vi "Security System.vi"() -> ()   [LabVIEW 2013]
doc: "This VI simulates the security system by monitoring the\n- Alarm switches\n- Bypass switches, \n-Tamper switches and indicates the corresponding activity with different colours.\nTHe system provides for one indicator light for each zone i.e.\n-Green: Normal\n-Red: Alarm\n-Blue: Bypass\n-Orange: Tamper.\n\n-A bypass input can override an alarm input but can not change the the existing condition of alarm\n-A Tamper input can override both alarm and bypass input but can not change the the existing condition of alarm and bypass.\n-An existing condition can be indicated when an override input is removed."
uses:
  Controls/Security System Indicators.ctl
  Controls/Security States.ctl
  Controls/FGV.ctl
  Controls/Write txt.ctl
panel:
  in  "stop simulation":bool
  out "Zone status indicators":T1
  in  "Tamper":bool[](array[boolean])
  in  "Bypass":bool[](array[boolean])
  in  "Alarm":bool[](array[boolean])
  # "· Green: Normal\n· Red: Alarm\n· Blue: Bypass\n· Orange: Tampe"
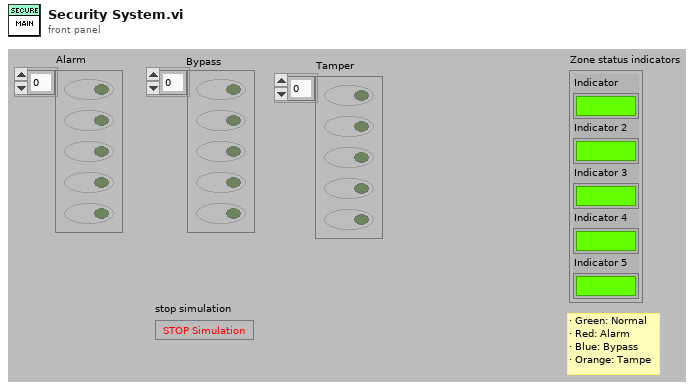
[diagram p1: front panel]
types:
  T1 = typedef "Security System Indicators.ctl" = cluster{"Indicator":bool, "Indicator 2":bool, "Indicator 3":bool, "Indicator 4":bool, "Indicator 5":bool}
  T2 = typedef "Security States.ctl" = enum16{"Initialize", "Main", "Stop"}
  T3 = typedef "Write txt.ctl" = enum16{"Initialize", "Write", "Stop"}
  T4 = typedef "FGV.ctl" = enum16{"Set", "Get"}
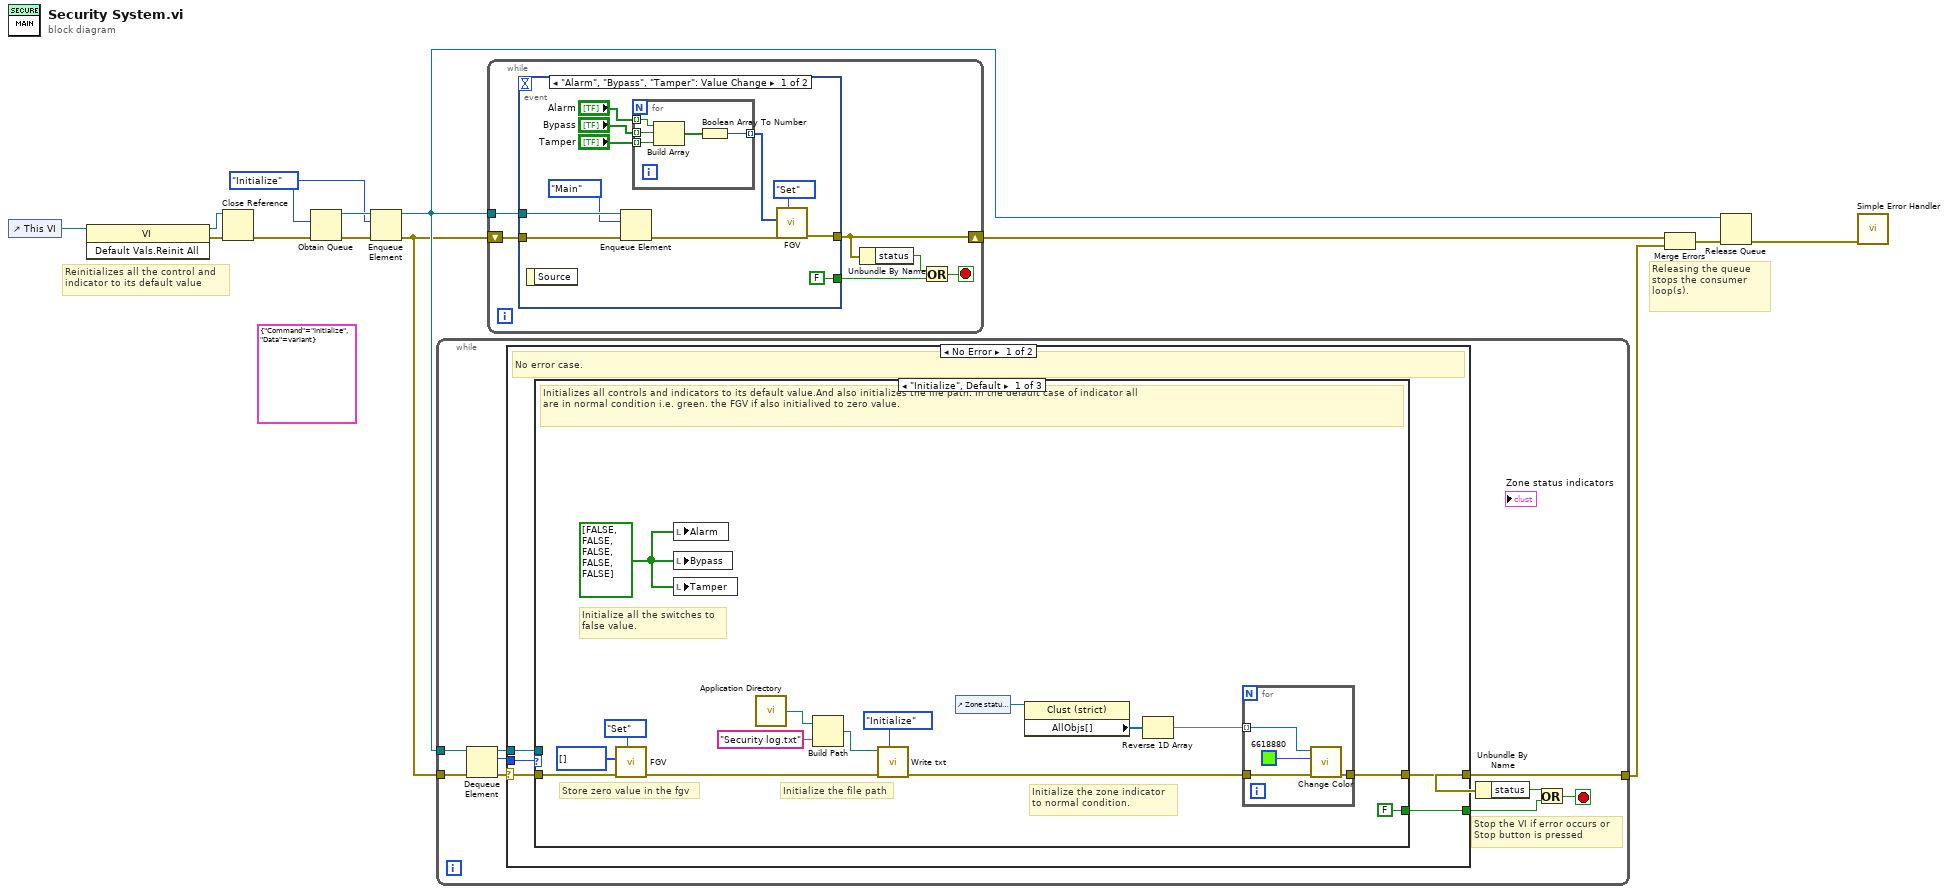
[diagram p0: block diagram]
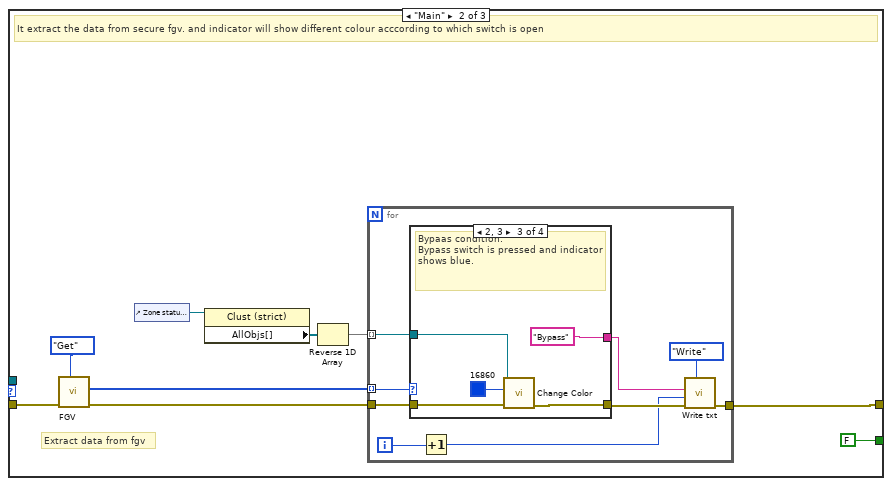
[diagram p2: hidden frame]
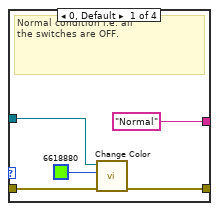
[diagram p3: hidden frame]
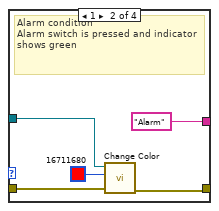
[diagram p4: hidden frame]
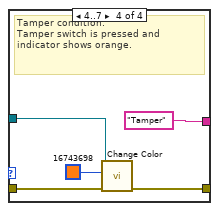
[diagram p5: hidden frame]
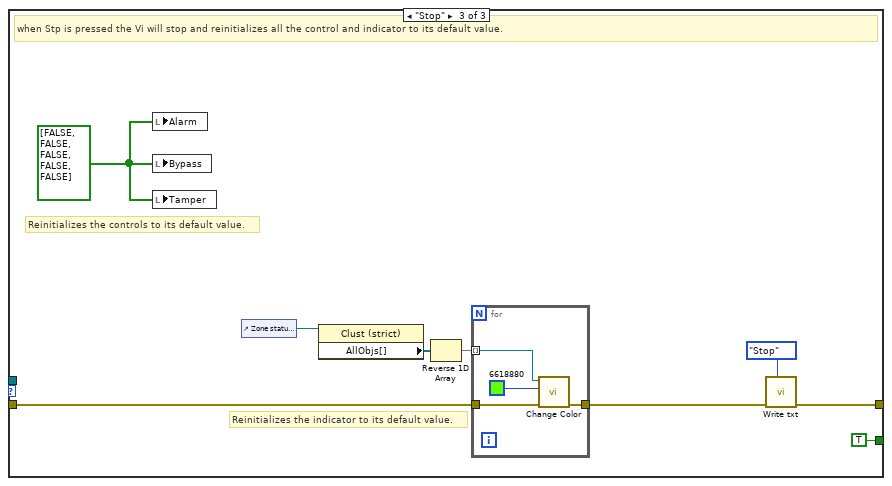
[diagram p6: hidden frame]
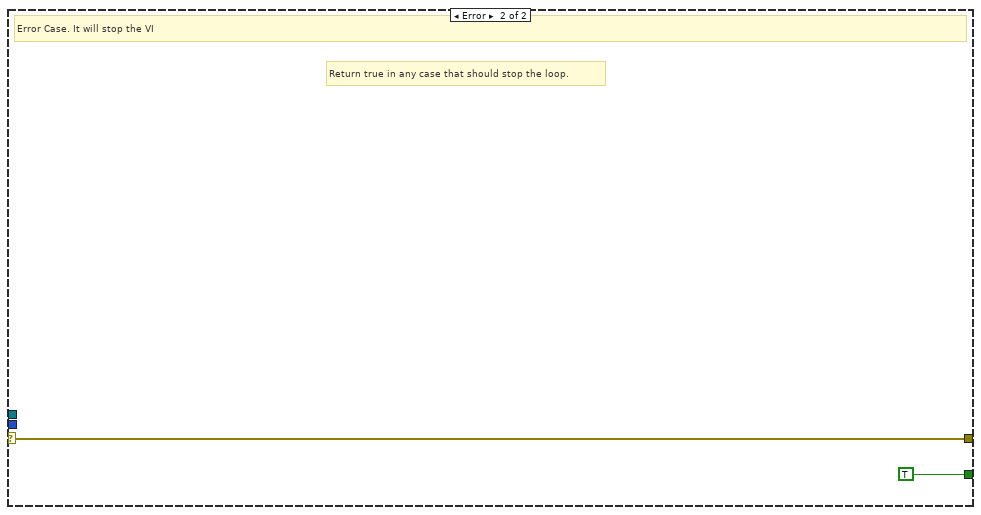
[diagram p7: hidden frame]
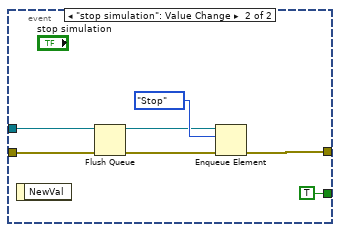
[diagram p8: hidden frame]
diagram:
  (unwired) cluster{"Command":T2, "Data":variant} {"Command"=enum."Initialize", "Data"=variant}
  w9 = Security_States."Initialize" ("Command")
  # "Reinitializes all the control and \nindicator to its default value"
  # "Releasing the queue stops the consumer loop(s)."
  n1 = control-ref of="This VI"() -> (w8:refnum<vi>)
  n2 = invoke class="VI" method="Default Vals.Reinit All"(reference=w8) -> (reference out=w6:refnum<vi>, error out=w7:errorcluster)  [unwired: 2 in, 1 out]
  n3 = Close Reference(reference=w6, error in (no error)=w7) -> (error out=w5:errorcluster)
  n4 = Obtain Queue(element data type=w9, error in (no error)=w5) -> (queue out=w12:refnum<queue>, error out=w11:errorcluster)  [unwired: 3 in, 1 out]
  n5 = Enqueue Element(queue=w12, element=w9, error in (no error)=w11) -> (queue out=w10:refnum<queue>, error out=w4:errorcluster)  [unwired: 1 in, 1 out]
  n6 = while {
    tunnel: w10 -> [w22]
    tunnel: w4 -> [w14]
    tunnel: [w19] -> w2
    stop <- w17 stop-if-true
    # "Stop the VI if error occurs or\nStop button is pressed"
    n7 = Dequeue Element(queue=w22, error in (no error)=w14) -> (queue out=w16:refnum<queue>, element=w20:T2, error out=w21:errorcluster)  [unwired: 1 in, 1 out]
    n8 = case shown="No Error" w21 {
      selector: w21 -> [w26 w99]
      tunnel: w20 -> [w25 _]
      tunnel: [w27 w99] -> w19
      tunnel: w16 -> [w24 _]
      tunnel: [w23 TRUE] -> w15
      frame No Error {
        # "No error case."
        n9 = case shown="\"Initialize\", Default" w25 {
          tunnel: [w34 w47 w86] -> w27
          tunnel: w26 -> [w42 w55 w88]
          tunnel: w24 -> [_ _ _]
          tunnel: [FALSE FALSE TRUE] -> w23
          frame "Initialize", Default {
            w36 = bool[] [FALSE, FALSE, FALSE, FALSE, FALSE] ("Alarm")
            # "Initialize all the switches to \nfalse value."
            # "Initialize the zone indicator \nto normal condition."
            # "Initialize the file path"
            # "Store zero value in the fgv"
            # "Initializes all controls and indicators to its default value.And also initializes the file path. In the default case of indicator all \nare in normal condition i.e. green. the FGV if also initialived to zero value."
            n10 = call "FGV.vi"("Enum"=FGV."Set", "error in (no error)"=w42, "Array"=u32[] [] ("Number in")) -> ("error out"=w33:errorcluster)  [unwired: 7 in, 1 out]
            n11 = local write "Alarm"(w36) -> ()
            n12 = local write "Bypass"(w36) -> ()
            n13 = local write "Tamper"(w36) -> ()
            n14 = call <vilib>:"Application Directory.vi"() -> ("Application Directory"=w30:path)
            n15 = Build Path(base path=w30, name or relative path="Security log.txt") -> (appended path=w29:path)
            n16 = call "Write txt.vi"("Enum"=Write_txt."Initialize", "error in"=w33, "file path"=w29) -> ("error out"=w32:errorcluster)  [unwired: 8 in]
            n17 = control-ref of="Zone status indicators"() -> (w38:refnum<vi>)
            n18 = property on="Property Node" class="Clust (strict)"(reference=w38) -> ("AllObjs[]"=w37:refnum<vi>[])  [unwired: 1 in, 2 out]
            n19 = Reverse 1D Array(array=w37) -> (reversed array=w35:refnum<vi>[])
            n20 = for {
              tunnel: w35 -> [w46] mode=indexing
              tunnel: w32 -> [w44]
              tunnel: [w43] -> w34
              n21 = call "Change Color.vi"("error in (no error)"=w44, "Color Box"=u32 6618880, "GObject in"=w46) -> ("error out"=w43:errorcluster)  [unwired: 8 in]
            }
          }
          frame "Main" {
            # "Extract data from fgv"
            # "It extract the data from secure fgv. and indicator will show different colour acccording to which switch is open"
            n22 = call "FGV.vi"("Enum"=FGV."Get", "error in (no error)"=w55) -> ("error out"=w48:errorcluster, "Array 2"=w53:u32[])  [unwired: 8 in]
            n23 = control-ref of="Zone status indicators"() -> (w51:refnum<vi>)
            n24 = property on="Property Node" class="Clust (strict)"(reference=w51) -> ("AllObjs[]"=w50:refnum<vi>[])  [unwired: 1 in, 2 out]
            n25 = Reverse 1D Array(array=w50) -> (reversed array=w49:refnum<vi>[])
            n26 = for {
              tunnel: w53 -> [w64] mode=indexing
              tunnel: w49 -> [w63] mode=indexing
              tunnel: w48 -> [w62]
              tunnel: [w59] -> w47
              i -> [w61]
              n27 = case shown="2, 3" w64 {
                tunnel: w63 -> [w69 w74 w79 w84]
                tunnel: w62 -> [w67 w72 w77 w82]
                tunnel: [w66 w71 w76 w81] -> w60
                tunnel: ["Normal" "Alarm" "Bypass" "Tamper"] -> w58
                frame 0, Default {
                  # "Normal condition i.e. all \nthe switches are OFF."
                  n28 = call "Change Color.vi"("error in (no error)"=w67, "Color Box"=u32 6618880, "GObject in"=w69) -> ("error out"=w66:errorcluster)  [unwired: 8 in]
                }
                frame 1 {
                  # "Alarm condition\nAlarm switch is pressed and indicator shows green"
                  n29 = call "Change Color.vi"("error in (no error)"=w72, "Color Box"=u32 16711680, "GObject in"=w74) -> ("error out"=w71:errorcluster)  [unwired: 8 in]
                }
                frame 2, 3 {
                  # "Bypaas condition.\nBypass switch is pressed and indicator shows blue."
                  n30 = call "Change Color.vi"("error in (no error)"=w77, "Color Box"=u32 16860, "GObject in"=w79) -> ("error out"=w76:errorcluster)  [unwired: 8 in]
                }
                frame 4..7 {
                  # "Tamper condition.\nTamper switch is pressed and indicator shows orange."
                  n31 = call "Change Color.vi"("error in (no error)"=w82, "Color Box"=u32 16743698, "GObject in"=w84) -> ("error out"=w81:errorcluster)  [unwired: 8 in]
                }
              }
              n32 = Increment(x=w61) -> (x+1=w57:i32)
              n33 = call "Write txt.vi"("Enum"=Write_txt."Write", "error in"=w60, "Zone"=w57, "Status"=w58) -> ("error out"=w59:errorcluster)  [unwired: 7 in]
            }
          }
          frame "Stop" {
            w89 = bool[] [FALSE, FALSE, FALSE, FALSE, FALSE] ("Alarm")
            # "Reinitializes the controls to its default value."
            # "Reinitializes the indicator to its default value."
            # "when Stp is pressed the Vi will stop and reinitializes all the control and indicator to its default value."
            n34 = local write "Alarm"(w89) -> ()
            n35 = local write "Bypass"(w89) -> ()
            n36 = local write "Tamper"(w89) -> ()
            n37 = control-ref of="Zone status indicators"() -> (w91:refnum<vi>)
            n38 = property on="Property Node" class="Clust (strict)"(reference=w91) -> ("AllObjs[]"=w92:refnum<vi>[])  [unwired: 1 in, 2 out]
            n39 = Reverse 1D Array(array=w92) -> (reversed array=w90:refnum<vi>[])
            n40 = for {
              tunnel: w90 -> [w97] mode=indexing
              tunnel: w88 -> [w95]
              tunnel: [w94] -> w87
              n41 = call "Change Color.vi"("error in (no error)"=w95, "Color Box"=u32 6618880, "GObject in"=w97) -> ("error out"=w94:errorcluster)  [unwired: 8 in]
            }
            n42 = call "Write txt.vi"("Enum"=Write_txt."Stop", "error in"=w87) -> ("error out"=w86:errorcluster)  [unwired: 9 in]
          }
        }
      }
      frame Error {
        # "Return true in any case that should stop the loop."
        # "Error Case. It will stop the VI"
      }
    }
    n43 = Unbundle By Name(w19) -> ("status"=w18:bool)
    n44 = Or(x=w18, y=w15) -> (x .or. y?=w17:bool)
  }
  n45 = while {
    shift-right: [w101] -> w13
    shift-left: w4 -> [w104]
    tunnel: w10 -> [w105]
    stop <- w102 stop-if-true
    n46 = event shown="[0] \"Alarm\", \"Bypass\", \"Tamper\": Value Change" {
      selector: _ -> [_ _]
      dyn-events: _ -> [_ _]
      timeout: _ -> [_ _]
      tunnel: w105 -> [w107 w125]
      tunnel: w104 -> [w112 w127]
      tunnel: [w113 w126] -> w101
      tunnel: [FALSE ("stop") TRUE ("stop")] -> w103
      event "Alarm", "Bypass", "Tamper": Value Change {
        n47 = event-data() -> ()  [unwired: 1 in, 1 out]
        n48 = Enqueue Element(queue=w107, element=Security_States."Main", error in (no error)=w112) -> (error out=w108:errorcluster)  [unwired: 1 in, 2 out]
        n49 = for {
          tunnel: "Alarm" -> [w121] mode=indexing
          tunnel: "Bypass" -> [w120] mode=indexing
          tunnel: "Tamper" -> [w119] mode=indexing
          tunnel: [w117] -> w110 mode=indexing
          n50 = Build Array(w121, w120, w119) -> (w118:bool[])
          n51 = Boolean Array To Number(Boolean array=w118) -> (number=w117:u32)
        }
        n52 = call "FGV.vi"("Enum"=FGV."Set", "error in (no error)"=w108, "Array"=w110) -> ("error out"=w113:errorcluster)  [unwired: 7 in, 1 out]
      }
      event "stop simulation": Value Change {
        n53 = event-data() -> ()  [unwired: 1 in, 1 out]
        n54 = Flush Queue(queue=w125) -> (queue out=w122:refnum<queue>)  [unwired: 1 in, 2 out]
        n55 = Enqueue Element(queue=w122, element=Security_States."Stop", error in (no error)=w127) -> (error out=w126:errorcluster)  [unwired: 1 in, 2 out]
      }
    }
    n56 = Unbundle By Name(w101) -> ("status"=w100:bool)
    n57 = Or(x=w100, y=w103) -> (x .or. y?=w102:bool)
  }
  n58 = Merge Errors(w13, w2) -> (w3:errorcluster)
  n59 = Release Queue(queue=w10, error in (no error)=w3) -> (error out=w1:errorcluster)  [unwired: 1 in, 2 out]
  n60 = call <vilib>:"Simple Error Handler.vi"("error in (no error)"=w1) -> ()  [unwired: 4 in, 5 out]
